vi "ini Ctrl_Var.vi"(5 "데이터타입":enum16{"I16", "U32", "경로"}(ring), 7 "Select":enum16{"Save", "Load"}(ring), 8 "에러 입력":errorcluster caption="에러 입력(에러 없음)", 9 "값":variant, 10 "키":string, 11 "섹션":string) -> (0 "에러 출력":errorcluster, 1 "값":string, 2 "경로 출력":path)   [LabVIEW 2020]
uses:
  Controls/Cmd_File path.ctl
  Controls/Cmd_File Type.ctl
  <vilib>/Utility/config.llb/Write Key (String).vi
  <vilib>/Utility/config.llb/Read Key (String).vi
  <vilib>/Utility/config.llb/NI_LVConfig.lvlib
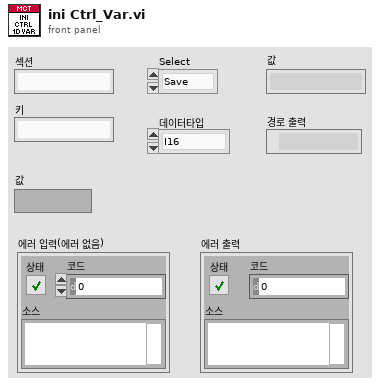
[diagram p1: front panel]
types:
  T1 = typedef "Cmd_File Type.ctl" = enum16{"엑셀", "엑셀(2003)", "텍스트", "설정", "2진", "VI", "CSV", "LOG", "폴더"}
  T2 = typedef "Cmd_File path.ctl" = enum16{"에러로그", "데이터파일경로", "성적서원본", "지난성적서", "Data Files", "경로생성", "Updater", "Template", "설정파일경로", "FTP Upload", "Update 경로", "어플리케이션"}
  T3 = typedef "NI_LVConfig.lvlib/Config Data RefNum.ctl" = refnum<k1>
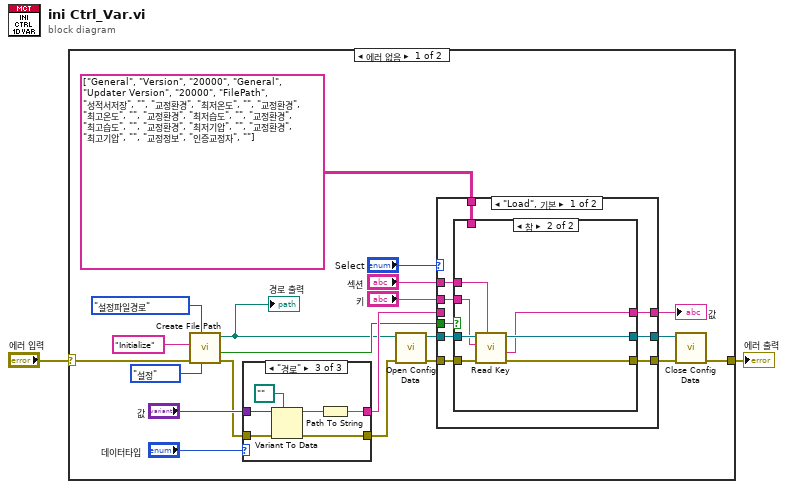
[diagram p0: block diagram]
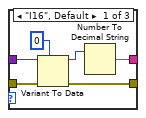
[diagram p2: hidden frame]
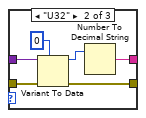
[diagram p3: hidden frame]
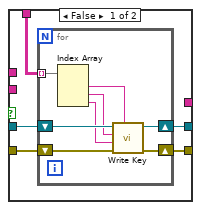
[diagram p4: hidden frame]
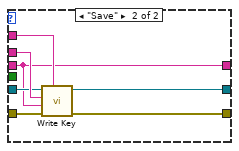
[diagram p5: hidden frame]
diagram:
  n1 = case shown="에러 없음" "에러 입력" {
    selector: "에러 입력" -> [w15 w78]
    tunnel: [w11 w78] -> w2
    frame No Error {
      n2 = call "Create File Path.vi"("파일타입"=Cmd_File_Type."설정", "항목"=Cmd_File_path."설정파일경로", "에러 입력"=w15, "문자열 in"="Initialize") -> ("error out"=w14:errorcluster, "파일존재?"=w13:bool, "파일경로"=w8:path)  [unwired: 4 in, 1 out]
      "경로 출력" <- w8
      n3 = case shown="\"경로\"" "데이터타입" {
        tunnel: "값" -> [w28 w34 w40]
        tunnel: w14 -> [w29 w35 w41]
        tunnel: [w27 w33 w39] -> w9
        tunnel: [w25 w31 w36] -> w19
        frame "I16", Default {
          n4 = Variant To Data(error in=w29, type=i16 0, Variant=w28) -> (data=w26:i16, error out=w27:errorcluster)
          n5 = Number To Decimal String(number=w26) -> (decimal integer string=w25:string)  [unwired: 1 in]
        }
        frame "U32" {
          n6 = Variant To Data(error in=w35, type=u32 0, Variant=w34) -> (data=w32:u32, error out=w33:errorcluster)
          n7 = Number To Decimal String(number=w32) -> (decimal integer string=w31:string)  [unwired: 1 in]
        }
        frame "경로" {
          n8 = Variant To Data(error in=w41, type=path "", Variant=w40) -> (data=w37:path, error out=w39:errorcluster)
          n9 = Path To String(path=w37) -> (string=w36:string)
        }
      }
      n10 = call <vilib>:"Open Config Data.vi"("error in (no error)"=w9, "configuration file path"=w8) -> ("error out"=w6:errorcluster, "refnum"=w7:T3)  [unwired: 7 in, 1 out]
      n11 = case shown="\"Load\", 기본" "Select" {
        tunnel: [w48 w77] -> w12
        tunnel: "키" -> [w45 w76]
        tunnel: "섹션" -> [w46 w75]
        tunnel: w6 -> [w50 w74]
        tunnel: w7 -> [w49 w73]
        tunnel: w13 -> [w47 _]
        tunnel: string[][] [["General", "Version", "20000"], ["General", "Updater Version", "20000"], ["FilePath", "성적서저장", ""], ["교정환경", "최저온도", ""], ["교정환경", "최고온도", ""], ["교정환경", "최저습도", ""], ["교정환경", "최고습도", ""], ["교정환경", "최저기압", ""], ["교정환경", "최고기압", ""], ["교정정보", "인증교정자", ""]] -> [w44 _]
        tunnel: w19 -> [_ w71]
        tunnel: [w43 w72] -> w10
        tunnel: [w42 w71] -> w5
        frame "Load", Default {
          n12 = case shown="참" w47 {
            tunnel: w50 -> [w52 w70]
            tunnel: w49 -> [w51 w69]
            tunnel: [w55 w66] -> w48
            tunnel: w46 -> [_ w68]
            tunnel: w45 -> [_ w67]
            tunnel: w44 -> [w54 _]
            tunnel: [w53 w65] -> w43
            tunnel: [_ w64] -> w42
            frame False {
              n13 = for {
                shift-right: [w60] -> w55
                shift-left: w52 -> [w63]
                shift-right: [w61] -> w53
                shift-left: w51 -> [w62]
                tunnel: w54 -> [w59] mode=indexing
                n14 = Index Array(array=w59) -> (element #1=w58:string, element #2=w57:string, element #3=w56:string)  [unwired: 3 in]
                n15 = call-poly <vilib>:"Write Key.vi"("section"=w58, "error in (no error)"=w63, "value"=w56, "key"=w57, "refnum"=w62) -> ("error out"=w60:errorcluster, "refnum out"=w61:T3)  [unwired: 4 in, 1 out]
              }
            }
            frame True {
              n16 = call-poly <vilib>:"Read Key.vi"("section"=w68, "error in (no error)"=w70, "key"=w67, "refnum"=w69) -> ("error out"=w66:errorcluster, "value"=w64:string, "refnum out"=w65:T3)  [unwired: 4 in, 1 out]
            }
          }
        }
        frame "Save" {
          n17 = call-poly <vilib>:"Write Key.vi"("section"=w75, "error in (no error)"=w74, "value"=w71, "key"=w76, "refnum"=w73) -> ("error out"=w77:errorcluster, "refnum out"=w72:T3)  [unwired: 4 in, 1 out]
        }
      }
      "값" <- w5
      n18 = call <vilib>:"Close Config Data.vi"("error in (no error)"=w12, "refnum"=w10) -> ("error out"=w11:errorcluster)  [unwired: 8 in, 1 out]
    }
    frame Error {
    }
  }
  "에러 출력" <- w2
